vi "Action setup.vi"(3 "Setup":T1[](array[typedef]) {"Private"."Offset" format="%^_3e"; "Private"."Scale Factors" format="%^_3e"}) -> (1 "Array":T1[](array[typedef]) {"Private"."Offset" format="%^_3e"; "Private"."Scale Factors" format="%^_3e"})   [LabVIEW 2021]
uses:
  New NML Data Acq/Sub Controls/Instrument Properties.ctl
  New NML Data Acq/Sub Controls/Public.ctl
  New NML Data Acq/Sub Controls/Private.ctl
  New NML Data Acq/Sub Controls/Instrument Ref.ctl
  New NML Data Acq/Sub Controls/SystemCheckBox-resize.ctl
panel:
  in  "Instrument Action":i32(listbox)
  in  "Delete":bool
  in  "Insert":bool
  out "Item Names":string[](array[string])
  in  "Done":bool
  in  "Configured Actions":i32(listbox)=2
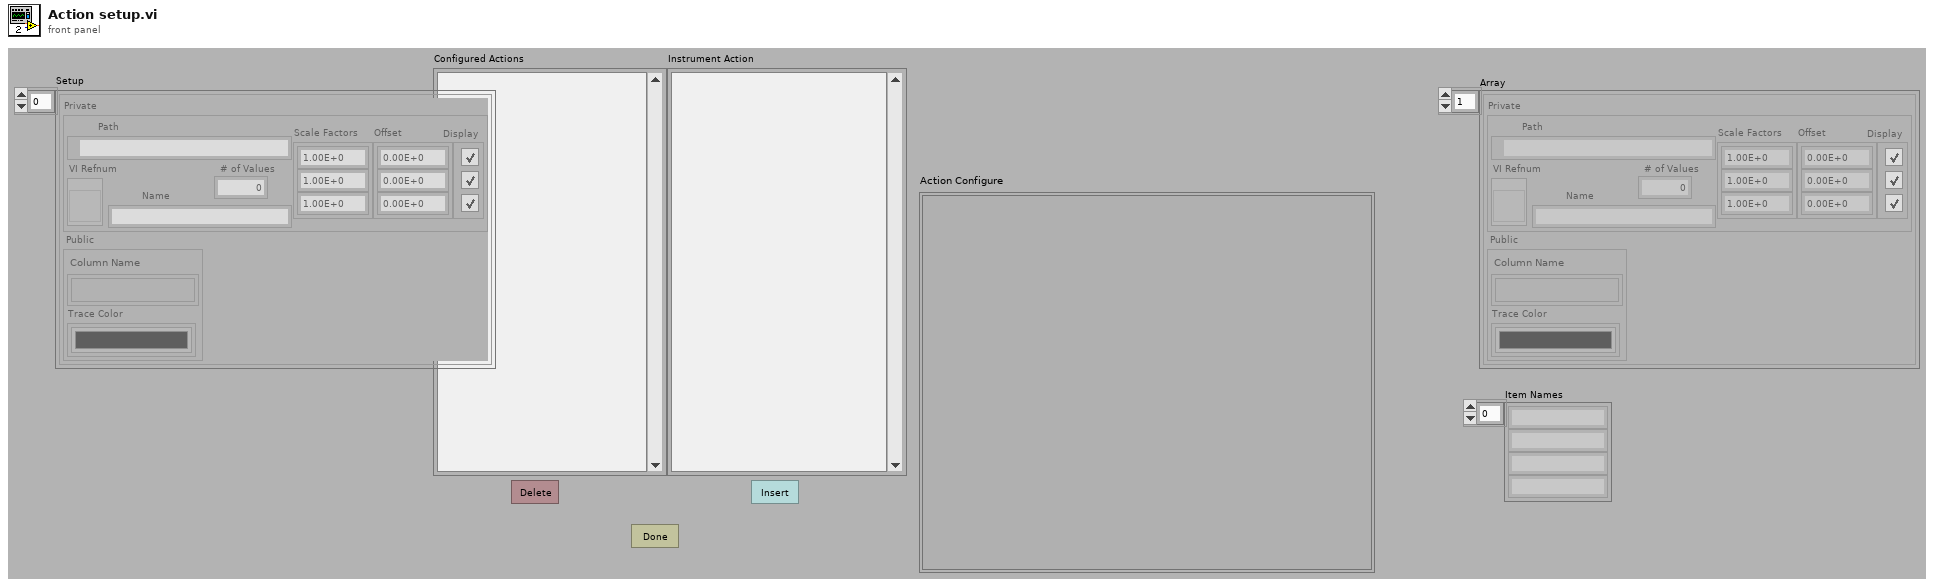
[diagram p1: front panel]
types:
  T1 = typedef "Instrument Properties.ctl" = cluster{"Public":T2, "Private":T3}
  T2 = typedef "Public.ctl" = cluster{"Column Name":string[], "Trace Color":u32[]}
  T3 = typedef "Private.ctl" = cluster{"Path":path, "VI Refnum":T4, "Name":string, "# of Values":i32, "Scale Factors":dbl[], "Display":T5[], "Offset":dbl[]}
  T4 = typedef "Instrument Ref.ctl" = refnum<vi>
  T5 = typedef "SystemCheckBox-resize.ctl" = bool
  T6 = typedef "Instrument Info.ctl" = cluster{"Name":string, "path":path}
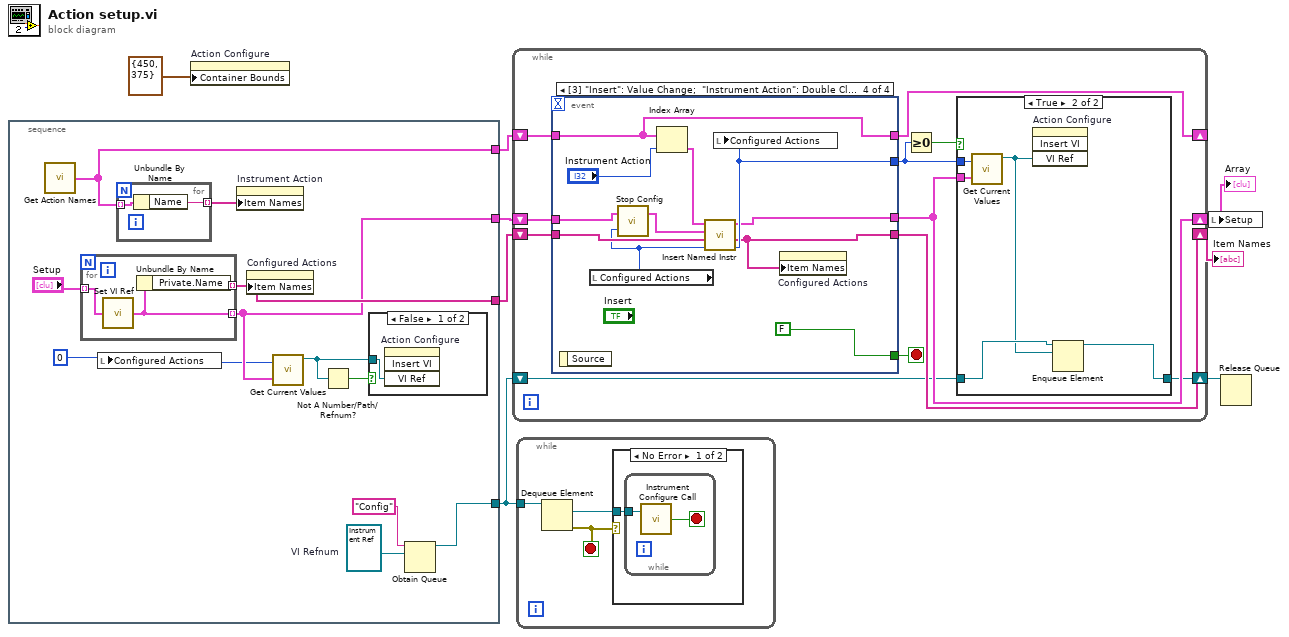
[diagram p0: block diagram]
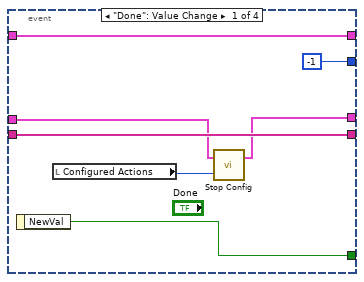
[diagram p5: hidden frame]
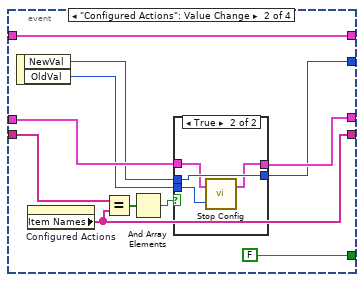
[diagram p6: hidden frame]
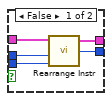
[diagram p7: hidden frame]
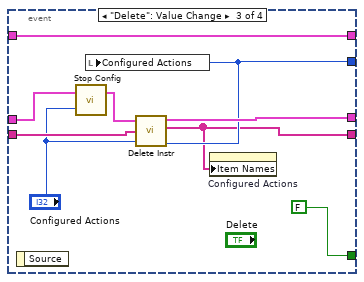
[diagram p8: hidden frame]
diagram:
  n1 = stacked-sequence {
    tunnel: [w15] -> w7
    tunnel: [w19] -> w6
    tunnel: [w16] -> w4
    tunnel: [w11] -> w2
    frame #0 {
      w12 = T4 refnum  # VI Refnum
      w14 = 0 ("Instrument List")
      n2 = call "Get Action Names.vi"() -> ("Names"=w16:T6[])  [unwired: 1 in]
      n3 = for {
        tunnel: "Setup" -> [w24] mode=indexing
        tunnel: [w25] -> w19 mode=indexing
        tunnel: [w23] -> w15 mode=indexing
        n4 = call "Set VI Ref.vi"("Instrument Prop In"=w24) -> ("Instrument Prop Out"=w23:T1)
        n5 = Unbundle By Name(w23) -> ("Private.Name"=w25:string)
      }
      n6 = local write "Configured Actions"(w14) -> ()
      n7 = for {
        tunnel: w16 -> [w22] mode=indexing
        tunnel: [w21] -> w17 mode=indexing
        n8 = Unbundle By Name(w22) -> ("Name"=w21:string)
      }
      n9 = property on="Instrument Action" class="LstBox (strict)"("Item Names"=w17) -> ()  [unwired: 2 in, 2 out]
      n10 = property on="Configured Actions" class="LstBox (strict)"("Item Names"=w19) -> ()  [unwired: 2 in, 2 out]
      n11 = call "Get Current Values.vi"("Instrument List"=w14, "Array"=w15) -> ("VI Ref"=w10:T4)  [unwired: 3 out]
      n12 = Not A Number/Path/Refnum?(number/path/refnum=w10) -> (NaN/Path/Refnum?=w9:bool)
      n13 = case shown="False" w9 {
        tunnel: w10 -> [w20 _]
        frame False {
          n14 = invoke on="Action Configure" class="SubPanel" method="Insert VI"("VI Ref"=w20) -> ()  [unwired: 3 in, 4 out]
        }
        frame True {
        }
      }
      n15 = Obtain Queue(name (unnamed)="Config", element data type=w12) -> (queue out=w11:refnum<queue>)  [unwired: 3 in, 2 out]
    }
  }
  n16 = property on="Action Configure" class="SubPnl"("Container Bounds"=cluster{"Width":u32, "Height":u32} {"Width"=450, "Height"=375} ("Bounds")) -> ()  [unwired: 2 in, 2 out]
  n17 = while {
    shift-right: [w32] -> w8
    shift-left: w7 -> [w35]
    shift-right: [w33] -> w5
    shift-left: w6 -> [w34]
    shift-right: [w28] -> _
    shift-left: w4 -> [w31]
    shift-right: [w26] -> w1
    shift-left: w2 -> [w27]
    stop <- w36 stop-if-true
    n18 = event shown="[3] \"Insert\": Value Change;  \"Instrument Action\": Double Click" {
      selector: _ -> [_ _ _ _]
      dyn-events: _ -> [_ _ _ _]
      timeout: _ -> [_ _ _ _]
      tunnel: [w48 FALSE ("Done") FALSE ("Done") FALSE ("Done")] -> w36
      tunnel: w35 -> [w44 w60 w71 w81]
      tunnel: [w43 w59 w76 w83] -> w32
      tunnel: w34 -> [w49 w51 w78 w89]
      tunnel: [w49 w52 w74 w79] -> w33
      tunnel: [-1 ("Instrument List Out") w55 w75 w84] -> w30
      tunnel: w31 -> [w46 w54 w73 w85]
      tunnel: [w46 w54 w73 w85] -> w28
      event "Done": Value Change {
        n19 = event-data() -> ("NewVal"=w48:bool)  [unwired: 1 in]
        n20 = local read "Configured Actions"() -> (w45:i32)
        n21 = call "Stop Config.vi"("OldVal"=w45, "Array"=w44) -> ("Array Out"=w43:T1[])  [unwired: 1 in]
      }
      event "Configured Actions": Value Change {
        n22 = event-data() -> ("NewVal"=w56:i32, "OldVal"=w58:i32)  [unwired: 1 in]
        n23 = property on="Configured Actions" class="LstBox (strict)"() -> ("Item Names"=w52:string[])  [unwired: 2 in, 2 out]
        n24 = Equal?(x=w51, y=w52) -> (x = y?=w53:bool[])
        n25 = And Array Elements(Boolean array=w53) -> (logical AND=w50:bool)
        n26 = case shown="True" w50 {
          tunnel: w60 -> [w65 w67]
          tunnel: [w64 w66] -> w59
          tunnel: w58 -> [w63 w68]
          tunnel: w56 -> [w62 w69]
          tunnel: [w61 w69] -> w55
          frame False {
            n27 = call "Rearrange Instr.vi"("Setup In"=w65, "NewVal"=w62, "OldVal"=w63) -> ("Setup Out"=w64:T1[], "NewVal Out"=w61:i32)  [unwired: 4 in]
          }
          frame True {
            n28 = call "Stop Config.vi"("OldVal"=w68, "Array"=w67) -> ("Array Out"=w66:T1[])  [unwired: 1 in]
          }
        }
      }
      event "Delete": Value Change {
        n29 = event-data() -> ()  [unwired: 1 in, 1 out]
        n30 = call "Stop Config.vi"("OldVal"="Configured Actions", "Array"=w71) -> ("Array Out"=w72:T1[])  [unwired: 1 in]
        n31 = call "Delete Instr.vi"("Setup"=w72, "Item Names"=w78, "Instrument List"="Configured Actions") -> ("Setup Out"=w76:T1[], "Item Names Out"=w74:string[], "Instrument List Out"=w75:i32)  [unwired: 1 in]
        n32 = local write "Configured Actions"(w75) -> ()
        n33 = property on="Configured Actions" class="LstBox (strict)"("Item Names"=w74) -> ()  [unwired: 2 in, 2 out]
      }
      event "Insert": Value Change; "Instrument Action": Double Click {
        n34 = event-data() -> ()  [unwired: 1 in, 1 out]
        n35 = local read "Configured Actions"() -> (w80:i32)
        n36 = call "Stop Config.vi"("OldVal"=w80, "Array"=w81) -> ("Array Out"=w82:T1[])  [unwired: 1 in]
        n37 = Index Array(array=w85, index="Instrument Action") -> (element=w86:T6)
        n38 = call "Insert Named Instr.vi"("new instrument"=w86, "Setup"=w82, "Configured Names"=w89, "Instrument List"=w80) -> ("dup Setup"=w83:T1[], "Item Names"=w79:string[], "Instrument List Out"=w84:i32)  [unwired: 2 in]
        n39 = local write "Configured Actions"(w84) -> ()
        n40 = property on="Configured Actions" class="LstBox (strict)"("Item Names"=w79) -> ()  [unwired: 2 in, 2 out]
      }
    }
    n41 = Greater Or Equal To 0?(x=w30) -> (x >= 0?=w29:bool)
    n42 = case shown="True" w29 {
      tunnel: w32 -> [_ w42]
      tunnel: w30 -> [_ w41]
      tunnel: w27 -> [w37 w40]
      tunnel: [w37 w38] -> w26
      frame False {
      }
      frame True {
        n43 = call "Get Current Values.vi"("Instrument List"=w41, "Array"=w42) -> ("VI Ref"=w39:T4)  [unwired: 3 out]
        n44 = invoke on="Action Configure" class="SubPanel" method="Insert VI"("VI Ref"=w39) -> ()  [unwired: 3 in, 4 out]
        n45 = Enqueue Element(queue=w40, element=w39) -> (queue out=w38:refnum<queue>)  [unwired: 2 in, 2 out]
      }
    }
  }
  "Item Names" <- w5
  "Array" <- w8
  n46 = while {
    tunnel: w2 -> [w92]
    stop <- w91 stop-if-true
    n47 = Dequeue Element(queue=w92) -> (element=w90:T4, error out=w91:errorcluster)  [unwired: 2 in, 2 out]
    n48 = case shown="No Error" w91 {
      tunnel: w90 -> [w93 _]
      frame No Error {
        n49 = while {
          tunnel: w93 -> [w95]
          stop <- w94 stop-if-true
          n50 = call "Instrument Configure Call.vi"("VI Refnum"=w95) -> ("Stop?"=w94:bool)  [unwired: 1 in, 2 out]
        }
      }
      frame Error {
      }
    }
  }
  n51 = local write "Setup"(w8) -> ()
  n52 = Release Queue(queue=w1) -> ()  [unwired: 2 in, 3 out]
